vi "JKISM++ Convert HexStr to Data.vi"(2 "HEX String":string) -> (7 "Variant":variant)   [LabVIEW 2014, in "JKI-State-Machine-Plus.lvlib"]
uses:
  JKI-State-Machine-Plus.lvlib
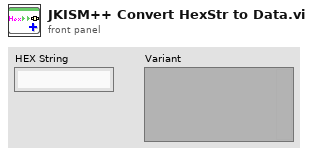
[diagram p1: front panel]
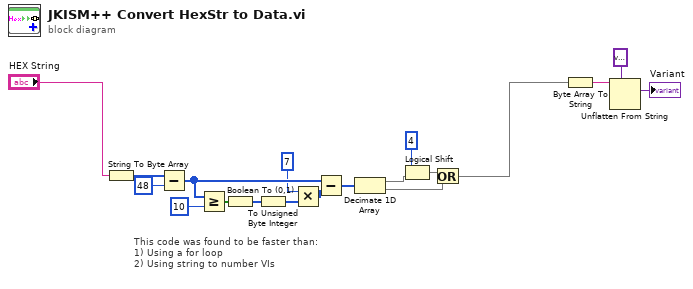
[diagram p0: block diagram]
diagram:
  # "This code was found to be faster than:\n1) Using a for loop\n2) Using string to number VIs"
  n1 = String To Byte Array(string="HEX String") -> (unsigned byte array=w3:u8[])
  n2 = Subtract(x=w3, y=u8 48) -> (x-y=w14:u8[])
  n3 = Greater Or Equal?(x=w14, y=u8 10) -> (x >= y?=w11:bool[])
  n4 = Boolean To (0,1)(Boolean=w11) -> (0, 1=w9:i16[])
  n5 = To Unsigned Byte Integer(number=w9) -> (unsigned 8bit integer=w12:u8[])
  n6 = Multiply(x=u8 7, y=w12) -> (x*y=w13:u8[])
  n7 = Subtract(x=w14, y=w13) -> (x-y=w5:u8[])
  n8 = Decimate 1D Array(w5) -> (w6:u8[], w4:u8[])
  n9 = Logical Shift(y=i8 4, x=w6) -> (x << y=w15:u8[])
  n10 = Or(x=w15, y=w4) -> (x .or. y?=w1:u8[])
  n11 = Byte Array To String(unsigned byte array=w1) -> (string=w17:string)
  n12 = Unflatten From String(type=variant, binary string=w17) -> (value=→"Variant":variant)  [unwired: 3 in, 2 out]
